vi "Create InstrumentStudio Plug-In.vi"() -> ()   [LabVIEW 2021, in "InstrumentStudio Plug-In Editor.lvlib"]
uses:
  _InstrumentStudio Plug-In Editor/InstrumentStudio Plug-In Editor.lvlib
  <vilib>/Utility/error.llb/ErrWarn.ctl
  _InstrumentStudio Plug-In Editor/controls/Data Holder.ctl
  _InstrumentStudio Plug-In Editor/NI_AB_API_PPL_Extensions/NI_AB_API_PPL_Extensions.lvclass
panel:
  in  "Group":string caption="InstrumentStudio Plug-in Group"
  out "Status":T1=TRUE caption="InstrumentStudio plug-in name must be unique and cannot contain any of the following characters:\n           \\ / : * ? \" < > |"
  in  "Create InstrumentStudio Plug-in":bool
  in  "Name":string caption="InstrumentStudio Plug-in Name"
  out "Active Project Name":string
  # "* Project in which the InstrumentStudio plug-in will be created"
  # "* Category under which the plug-in will be populated under\n   InstrumentStudio Edit Layout Dialog"
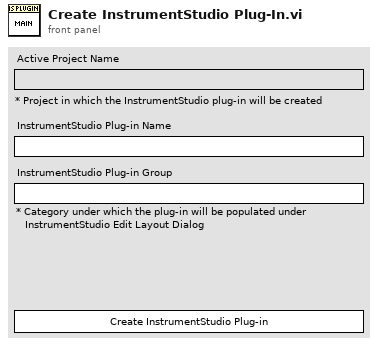
[diagram p1: front panel]
types:
  T1 = typedef "ErrWarn.ctl" = bool
  T2 = typedef "InstrumentStudio Plug-In Editor.lvlib/Data Holder.ctl" = cluster{"project ref":refnum<vi>, "Name":string, "Plugin Group Name":string}
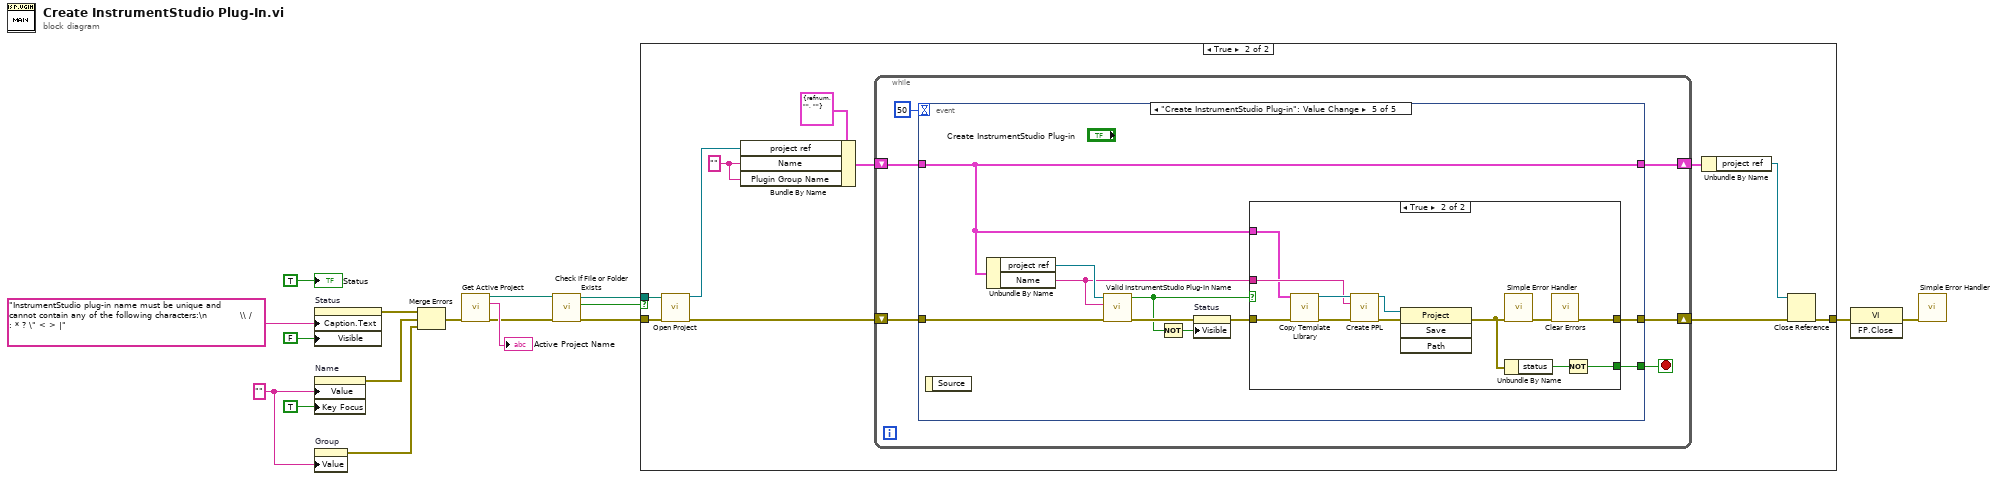
[diagram p0: block diagram]
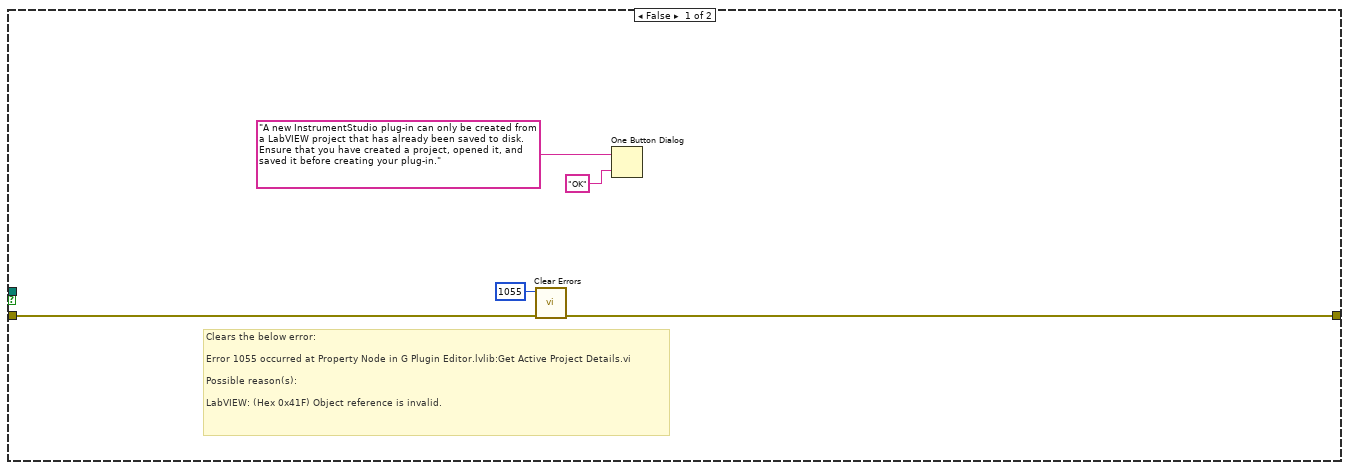
[diagram p2: hidden frame]
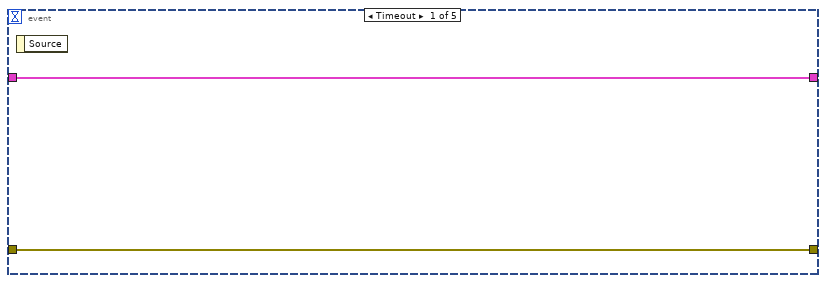
[diagram p3: hidden frame]
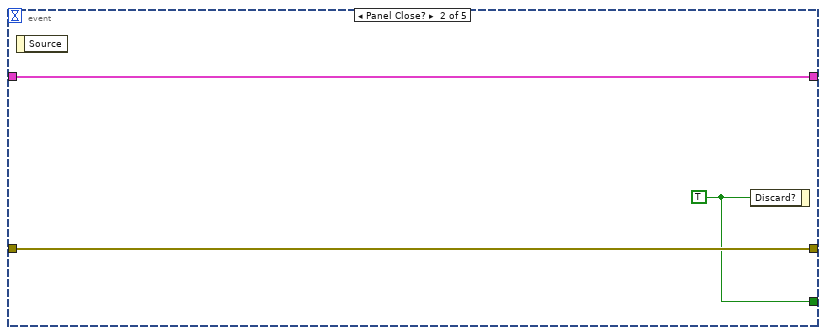
[diagram p4: hidden frame]
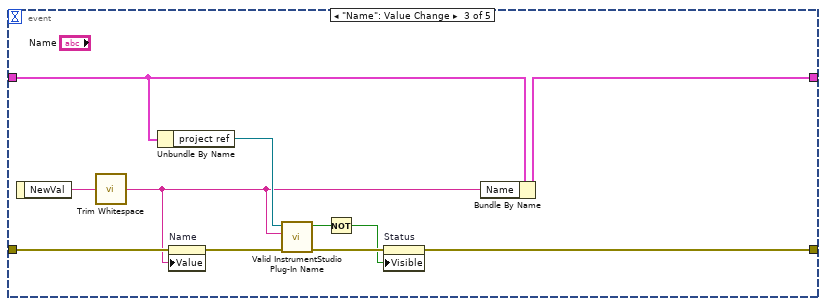
[diagram p5: hidden frame]
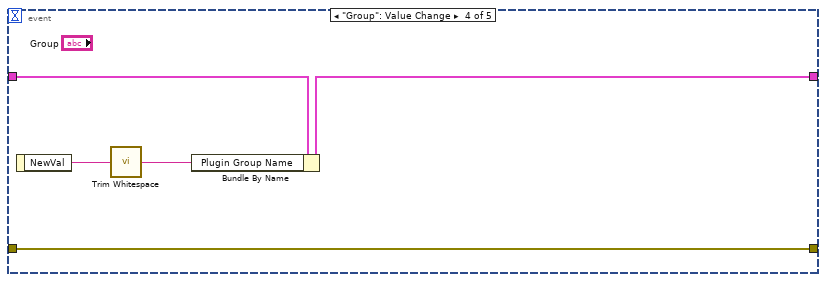
[diagram p6: hidden frame]
diagram:
  w1 = "" ("InstrumentStudio G Plug-in Name")
  n1 = property on="Status" class="Bool"("Caption.Text"="InstrumentStudio plug-in name must be unique and cannot contain any of the following characters:\n           \\ / : * ? \" < > |" ("Status"), "Visible"=FALSE) -> (error out=w14:errorcluster)  [unwired: 2 in, 1 out]
  n2 = property on="Name" class="Str"("Value"=w1, "Key Focus"=TRUE) -> (error out=w13:errorcluster)  [unwired: 2 in, 1 out]
  n3 = property on="Group" class="Str"("Value"=w1) -> (error out=w4:errorcluster)  [unwired: 2 in, 1 out]
  n4 = Merge Errors(w14, w13, w4) -> (w3:errorcluster)
  n5 = call "Get Active Project.vi"("error in"=w3) -> ("path"=w9:path, "name"=→"Active Project Name":string, "error out"=w2:errorcluster)  [unwired: 12 in]
  n6 = call <vilib>:"Check if File or Folder Exists.vi"("error in (no error)"=w2, "path"=w9) -> ("error out"=w10:errorcluster, "file or folder exists?"=w7:bool, "dup path"=w8:path)  [unwired: 7 in]
  n7 = case shown="True" w7 {
    tunnel: w10 -> [w20 w32]
    tunnel: [w19 w25] -> w11
    tunnel: w8 -> [_ w24]
    frame False {
      # "Clears the below error:\n\nError 1055 occurred at Property Node in G Plugin Editor.lvlib:Get Active Project Details.vi\n\nPossible reason(s):\n\nLabVIEW: (Hex 0x41F) Object reference is invalid."
      n8 = call <vilib>:"Clear Errors.vi"("error in (no error)"=w20, "specific error code to clear (0: all)"=1055) -> ("error out"=w19:errorcluster)  [unwired: 4 in, 1 out]
      n9 = One Button Dialog(message="A new InstrumentStudio plug-in can only be created from a LabVIEW project that has already been saved to disk.  Ensure that you have created a project, opened it, and saved it before creating your plug-in.", button name ("OK")="OK") -> ()  [unwired: 1 out]
    }
    frame True {
      w23 = "" ("Name")
      n10 = call "Open Project.vi"("path"=w24, "error in"=w32) -> ("project ref"=w30:refnum<vi>, "error out"=w33:errorcluster)  [unwired: 12 in]
      n11 = Bundle By Name(cluster=T2 {"project ref"=refnum, "Name"="", "Plugin Group Name"=""}, "project ref"=w30, "Name"=w23, "Plugin Group Name"=w23) -> (w29:T2)
      n12 = while {
        shift-right: [w36] -> w26
        shift-left: w33 -> [w39]
        shift-right: [w37] -> w28
        shift-left: w29 -> [w38]
        stop <- w34 stop-if-true
        n13 = event shown="[4] \"Create InstrumentStudio Plug-in\": Value Change" {
          selector: _ -> [_ _ _ _ _]
          dyn-events: _ -> [_ _ _ _ _]
          timeout: 50 -> [_ _ _ _ _]
          tunnel: w39 -> [w40 w43 w47 w59 w70]
          tunnel: w38 -> [w41 w44 w53 w60 w64]
          tunnel: [w41 w44 w54 w58 w64] -> w37
          tunnel: [w40 w43 w51 w59 w67] -> w36
          tunnel: [_ w42 _ _ w61] -> w34
          event Timeout {
            n14 = event-data() -> ()  [unwired: 1 in, 1 out]
          }
          event Panel Close? {
            w42 = TRUE ("Discard?")
            n15 = event-data() -> ()  [unwired: 1 in, 1 out]
            n16 = event-data("Discard?"=w42) -> ()  [unwired: 1 in, 1 out]
          }
          event "Name": Value Change {
            n17 = event-data() -> ("NewVal"=w55:string)  [unwired: 1 in]
            n18 = call <vilib>:"Trim Whitespace.vi"("string"=w55) -> ("trimmed string"=w46:string)  [unwired: 1 in]
            n19 = Unbundle By Name(w53) -> ("project ref"=w52:refnum<vi>)
            n20 = property on="Name" class="Str"(error in=w47, "Value"=w46) -> (error out=w48:errorcluster)  [unwired: 1 in, 1 out]
            n21 = call "Valid InstrumentStudio Plug-In Name.vi"("error in"=w48, "requested plugin name"=w46, "project ref"=w52) -> ("error out"=w50:errorcluster, "valid name?"=w45:bool)  [unwired: 7 in]
            n22 = Not(x=w45) -> (.not. x?=w49:bool)
            n23 = property on="Status" class="Bool"(error in=w50, "Visible"=w49) -> (error out=w51:errorcluster)  [unwired: 1 in, 1 out]
            n24 = Bundle By Name(cluster=w53, "Name"=w46) -> (w54:T2)
          }
          event "Group": Value Change {
            n25 = event-data() -> ("NewVal"=w57:string)  [unwired: 1 in]
            n26 = call <vilib>:"Trim Whitespace.vi"("string"=w57) -> ("trimmed string"=w56:string)  [unwired: 1 in]
            n27 = Bundle By Name(cluster=w60, "Plugin Group Name"=w56) -> (w58:T2)
          }
          event "Create InstrumentStudio Plug-in": Value Change {
            n28 = event-data() -> ()  [unwired: 1 in, 1 out]
            n29 = Unbundle By Name(w64) -> ("project ref"=w66:refnum<vi>, "Name"=w65:string)
            n30 = call "Valid InstrumentStudio Plug-In Name.vi"("error in"=w70, "requested plugin name"=w65, "project ref"=w66) -> ("error out"=w69:errorcluster, "valid name?"=w63:bool)  [unwired: 7 in]
            n31 = Not(x=w63) -> (.not. x?=w62:bool)
            n32 = property on="Status" class="Bool"(error in=w69, "Visible"=w62) -> (error out=w68:errorcluster)  [unwired: 1 in, 1 out]
            n33 = case shown="True" w63 {
              tunnel: w68 -> [w71 w83]
              tunnel: [w71 w75] -> w67
              tunnel: w65 -> [_ w80]
              tunnel: [_ w73] -> w61
              tunnel: w64 -> [_ w77]
              frame False {
              }
              frame True {
                n34 = call "Copy Template Library.vi"("configuration"=w77, "error in"=w83) -> ("project ref out"=w82:refnum<vi>, "error out"=w81:errorcluster)  [unwired: 12 in]
                n35 = call "Create PPL.vi"("Project Refnum"=w82, "Plug-in name"=w80, "error in (no error)"=w81) -> ("project ref out"=w79:refnum<vi>, "error out"=w78:errorcluster)  [unwired: 10 in, 1 out]
                n36 = invoke class="Project" method="Save"(reference=w79, error in=w78) -> (error out=w72:errorcluster)  [unwired: 2 in, 3 out]
                n37 = call <vilib>:"Simple Error Handler.vi"("error in (no error)"=w72) -> ("error out"=w76:errorcluster)  [unwired: 4 in, 4 out]
                n38 = Unbundle By Name(w72) -> ("status"=w74:bool)
                n39 = call <vilib>:"Clear Errors.vi"("error in (no error)"=w76) -> ("error out"=w75:errorcluster)  [unwired: 5 in, 1 out]
                n40 = Not(x=w74) -> (.not. x?=w73:bool)
              }
            }
          }
        }
      }
      n41 = Unbundle By Name(w28) -> ("project ref"=w27:refnum<vi>)
      n42 = Close Reference(reference=w27, error in (no error)=w26) -> (error out=w25:errorcluster)
    }
  }
  n43 = invoke class="VI" method="FP.Close"(error in=w11) -> (error out=w12:errorcluster)  [unwired: 2 in, 2 out]
  n44 = call <vilib>:"Simple Error Handler.vi"("error in (no error)"=w12) -> ()  [unwired: 4 in, 5 out]
  "Status" <- T1 TRUE ("Status")
